vi "ABC Find Step - Copy.vi"(4 "UART":refnum<vi>, 5 "ComPort":refnum<visa-resource-name>, 6 "Data":refnum<vi>, 7 "DaqTask":refnum<k21>, 8 "ErrIn":errorcluster, 9 "DirSize":cluster{"Dir":T1, "Size":i32}, 11 "DataIn":dbl[](array[numeric])=[0.0]) -> (0 "ErrOut":errorcluster, 1 "FrontPos":dbl, 2 "BackPos":dbl, 3 "DataOut":dbl[](array[numeric]))   [LabVIEW 2020]
uses:
  <userlib>/Amira UART/Public/TypeDefs/AUART StepDir.ctl
  <vilib>/DAQmx/read.llb/DAQmx Read (Digital 1D Bool 1Chan 1Samp).vi
  <vilib>/DAQmx/miscellaneous.llb/DAQmx Fill In Error Info.vi
  <userlib>/Amira UART/Amira UART.lvclass
  <userlib>/KQD LabVIEW User/Serial/Serial.lvlib
panel:
  out "FrontSW":bool
  out "BackSW":bool
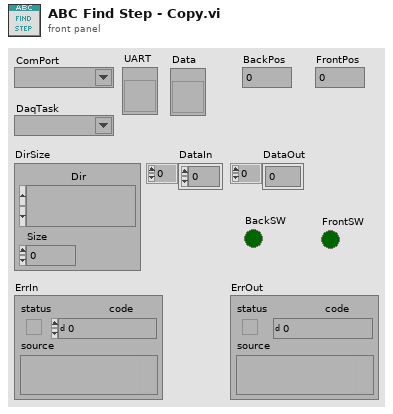
[diagram p1: front panel]
types:
  T1 = typedef "Amira UART.lvclass/AUART StepDir.ctl" = enum16{"", "compress", "decompress"}
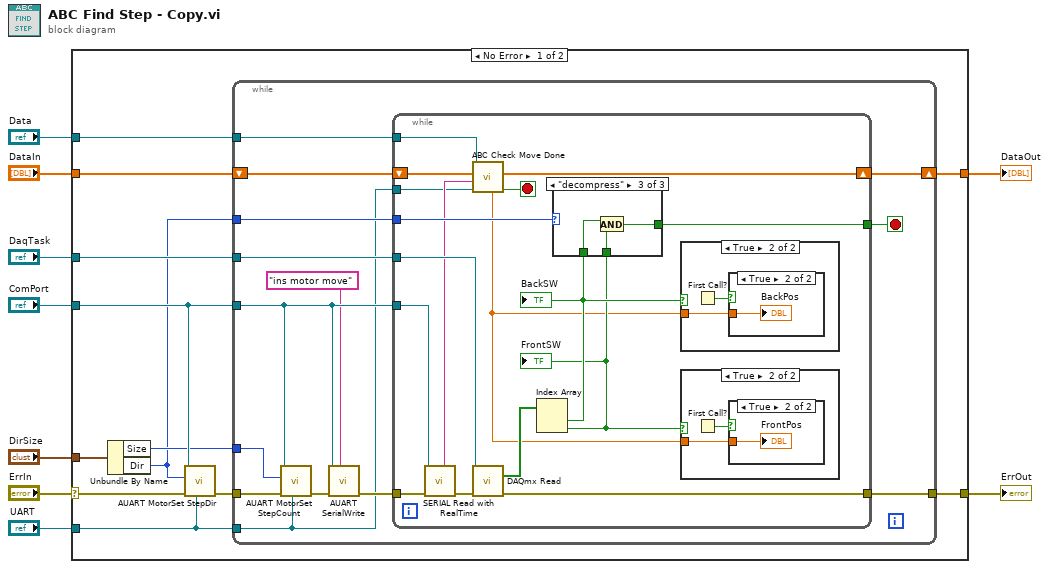
[diagram p0: block diagram]
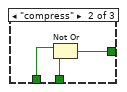
[diagram p7: hidden frame]
diagram:
  n1 = case shown="No Error" "ErrIn" {
    selector: "ErrIn" -> [w15 w65]
    tunnel: "UART" -> [w13 _]
    tunnel: "DaqTask" -> [w21 _]
    tunnel: [w20 w65] -> w7
    tunnel: "DataIn" -> [w19 w66]
    tunnel: [w18 w66] -> w5
    tunnel: "ComPort" -> [w16 _]
    tunnel: "DirSize" -> [w14 _]
    tunnel: "Data" -> [w11 _]
    frame No Error {
      n2 = Unbundle By Name(w14) -> ("Size"=w12:i32, "Dir"=w10:T1)
      n3 = call <userlib>:"AUART MotorSet StepDir.vi"("UART"=w13, "ErrIn"=w15, "step_dir"=w10, "Port"=w16) -> ("ErrOut"=w17:errorcluster)  [unwired: 7 in]
      n4 = while {
        tunnel: w21 -> [w31]
        tunnel: w16 -> [w25]
        tunnel: w13 -> [w22]
        tunnel: [w35] -> w20
        shift-right: [w27] -> w18
        shift-left: w19 -> [w33]
        tunnel: w17 -> [w30]
        tunnel: w12 -> [w29]
        tunnel: w11 -> [w28]
        tunnel: w10 -> [w26]
        stop <- w32 stop-if-true
        n5 = call <userlib>:"AUART MotorSet StepCount.vi"("UART"=w22, "ErrIn"=w30, "step_count"=w29, "Port"=w25) -> ("ErrOut"=w34:errorcluster)  [unwired: 7 in]
        n6 = call <userlib>:"AUART SerialWrite.vi"("Cmd"="ins motor move", "ErrIn"=w34, "Port"=w25) -> ("ErrOut"=w24:errorcluster)  [unwired: 7 in, 1 out]
        n7 = while {
          tunnel: [w51] -> w32
          tunnel: w31 -> [w50]
          tunnel: w28 -> [w43]
          tunnel: w26 -> [w49]
          tunnel: w25 -> [w48]
          shift-right: [w40] -> w27
          shift-left: w33 -> [w44]
          tunnel: w24 -> [w47]
          tunnel: [w45] -> w35
          tunnel: w22 -> [w41]
          stop <- w39 stop-if-true
          n8 = call <userlib>:"SERIAL Read with RealTime.vi"("ErrIn"=w47, "PortIn"=w48) -> ("ErrOut"=w46:errorcluster, "Response"=w42:string)  [unwired: 7 in, 1 out]
          n9 = call "ABC Check Move Done.vi"("UART"=w41, "Response"=w42, "DataIn"=w44, "Data"=w43) -> ("Done"=w39:bool, "DataOut"=w40:dbl[], "Position"=w36:dbl)  [unwired: 5 in]
          n10 = call-poly <vilib>:"DAQmx Read.vi"("task/channels in"=w50, "error in"=w46) -> ("data"=w52:bool[], "error out"=w45:errorcluster)  [unwired: 11 in, 1 out]
          n11 = Index Array(array=w52) -> (element #1=w38:bool, element #2=w37:bool)  [unwired: 2 in]
          "BackSW" <- w38
          "FrontSW" <- w37
          n12 = case shown="\"decompress\"" w49 {
            tunnel: [_ w61 w64] -> w51
            tunnel: w38 -> [_ w60 w63]
            tunnel: w37 -> [_ w59 w62]
            frame "", Default {
            }
            frame "compress" {
              n13 = Not Or(1:w59, 2:w60) -> (0:w61:bool)
            }
            frame "decompress" {
              n14 = And(x=w63, y=w62) -> (x .and. y?=w64:bool)
            }
          }
          n15 = case shown="True" w38 {
            tunnel: w36 -> [_ w56]
            frame False {
            }
            frame True {
              n16 = First Call?() -> (First Call?: T/F=w57:bool)
              n17 = case shown="True" w57 {
                tunnel: w56 -> [_ w58]
                frame False {
                }
                frame True {
                  "BackPos" <- w58
                }
              }
            }
          }
          n18 = case shown="True" w37 {
            tunnel: w36 -> [_ w53]
            frame False {
            }
            frame True {
              n19 = First Call?() -> (First Call?: T/F=w54:bool)
              n20 = case shown="True" w54 {
                tunnel: w53 -> [_ w55]
                frame False {
                }
                frame True {
                  "FrontPos" <- w55
                }
              }
            }
          }
        }
      }
    }
    frame Error {
    }
  }
  "ErrOut" <- w7
  "DataOut" <- w5
